vi "Trim String.vi"(1 "String In":string) -> (0 "String Out":string)   [LabVIEW 2021, in "Seq Edit Quick Drop.lvlib"]
uses:
  Seq Edit Quick Drop.lvlib
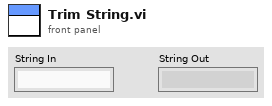
[diagram p1: front panel]
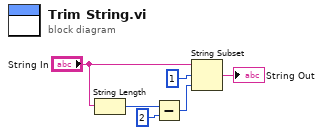
[diagram p0: block diagram]
diagram:
  n1 = String Length(string="String In") -> (length=w3:i32)
  n2 = Subtract(x=w3, y=2) -> (x-y=w5:i32)
  n3 = String Subset(string="String In", offset (0)=1, length (rest)=w5) -> (substring=→"String Out":string)
